vi "get.vi"(8 "error in (no error)":errorcluster, 10 "Parameter":string, 11 "dbm in":refnum<class "dbm.lvclass">) -> (0 "error out":errorcluster, 2 "Value":string, 3 "dbm out":refnum<class "dbm.lvclass">)   [LabVIEW 2013, in "dbm.lvclass"]
uses:
  dbm.lvclass
  dbm.lvclass/dbm.ctl
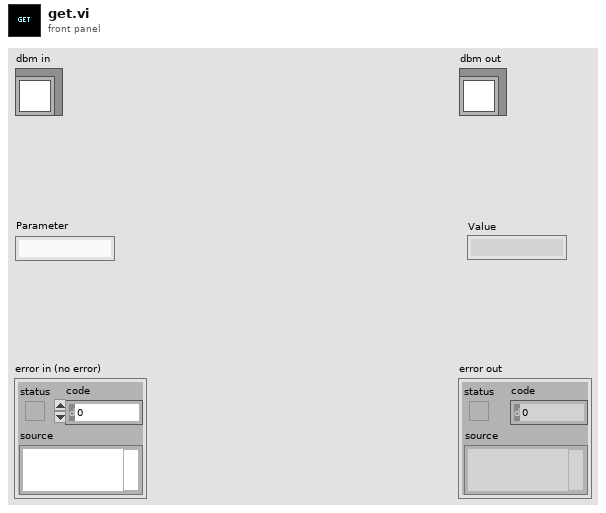
[diagram p1: front panel]
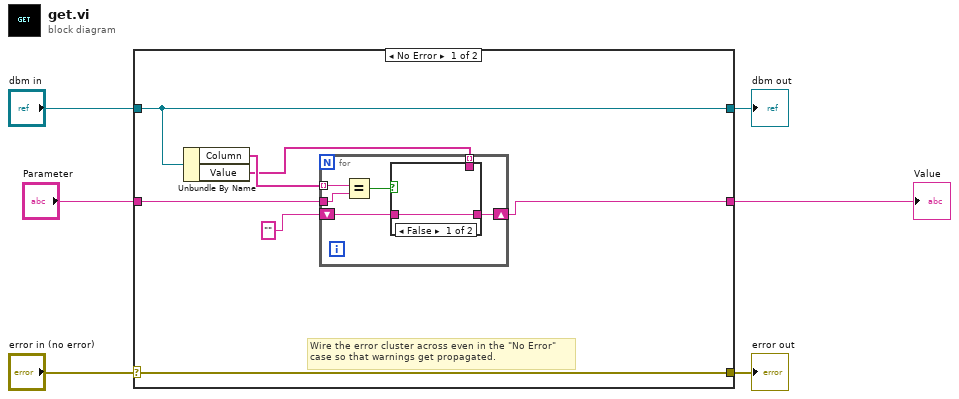
[diagram p0: block diagram]
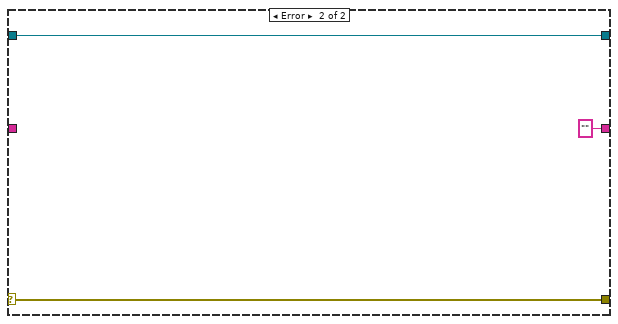
[diagram p3: hidden frame]
diagram:
  n1 = case shown="No Error" "error in (no error)" {
    selector: "error in (no error)" -> [w13 w24]
    tunnel: [w13 w24] -> w5
    tunnel: [w12 w23] -> w3
    tunnel: "dbm in" -> [w12 w23]
    tunnel: "Parameter" -> [w10 _]
    tunnel: [w8 "" ("Parameter")] -> w1
    frame No Error {
      # "Wire the error cluster across even in the \"No Error\"\ncase so that warnings get propagated."
      n2 = Unbundle By Name(w12) -> ("Column"=w11:string[], "Value"=w7:string[])
      n3 = for {
        tunnel: w11 -> [w19] mode=indexing
        tunnel: w10 -> [w18]
        shift-right: [w15] -> w8
        shift-left: "" -> [w16]
        tunnel: w7 -> [w14] mode=indexing
        n4 = Equal?(x=w19, y=w18) -> (x = y?=w17:bool)
        n5 = case shown="False" w17 {
          tunnel: w16 -> [w20 _]
          tunnel: [w20 w21] -> w15
          tunnel: w14 -> [_ w21]
          frame False {
          }
          frame True {
          }
        }
      }
    }
    frame Error {
    }
  }
  "error out" <- w5
  "dbm out" <- w3
  "Value" <- w1
